vi "GetEvent.vi"(7 "error in (no error)":errorcluster, 10 "reference in":refnum<class "DUT_Handler_Bailey.lvclass">) -> (0 "error out":errorcluster, 1 "Event":refnum<user-event>, 3 "reference in":refnum<class "DUT_Handler_Bailey.lvclass">)   [LabVIEW 2017]
uses:
  DUT_Handler_Bailey.lvclass
  Action.ctl
  EventData.ctl
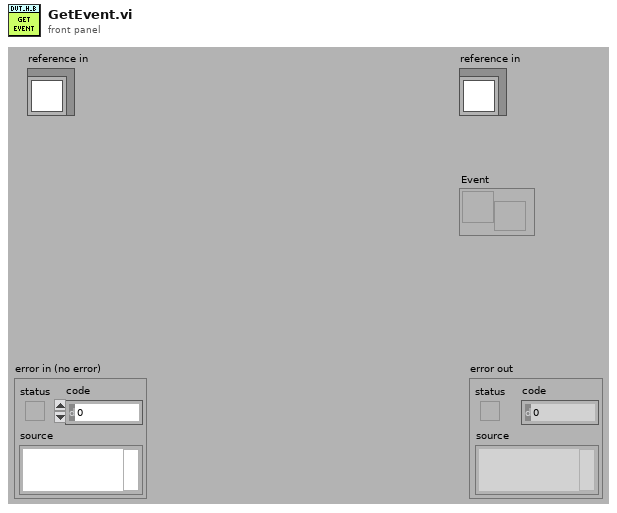
[diagram p1: front panel]
types:
  T1 = typedef "DUT_Handler_Bailey.lvlib/DUT_Handler_Bailey.lvclass/ObjectAttributes.ctl" = cluster{"Config":T2, "Barcode":refnum<class "Barcode_Reader_Base.lvclass">}
  T2 = typedef "DUT_Handler_Bailey.lvlib/DUT_Handler_Bailey.lvclass/Config.ctl" = cluster{"default":string}
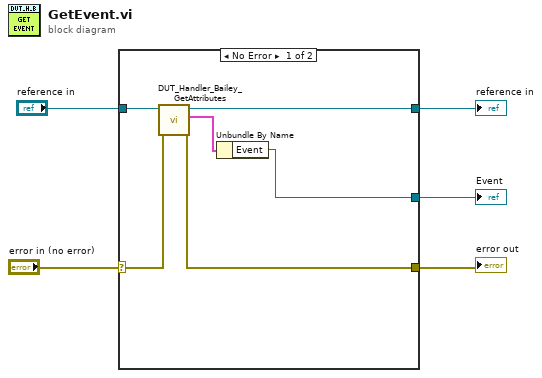
[diagram p0: block diagram]
diagram:
  n1 = case shown="No Error" "error in (no error)" {
    selector: "error in (no error)" -> [w11 w13]
    tunnel: [w9 w13] -> w4
    tunnel: [w7 w12] -> w2
    tunnel: "reference in" -> [w8 w12]
    tunnel: [w6 _] -> w1
    frame No Error {
      n2 = call "DUT_Handler_Bailey_GetAttributes.vi"("error in (no error)"=w11, "reference in"=w8) -> ("error out"=w9:errorcluster, "Data"=w10:T1, "reference out"=w7:refnum<class "DUT_Handler_Bailey.lvclass">)  [unwired: 6 in, 1 out]
      n3 = Unbundle By Name(w10) -> ("Event"=w6:refnum<user-event>)
    }
    frame Error {
    }
  }
  "error out" <- w4
  "reference in" <- w2
  "Event" <- w1
